vi "A_Read Set Pt Array.vi"(0 "Previous y":dbl, 1 "Period(ms)":dbl, 2 "Result":dbl, 5 "dt":u32, 7 "y array":dbl[](array[numeric]), 12 "arraysize":dbl, 13 "Integral in":dbl) -> (4 "Set Pt Out":dbl, 6 "Integral out":dbl)   [LabVIEW 2011]
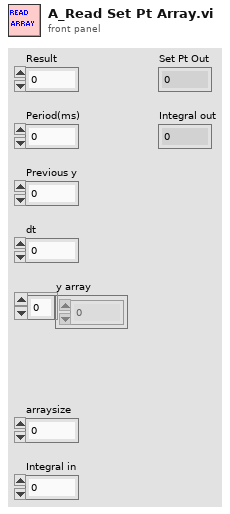
[diagram p1: front panel]
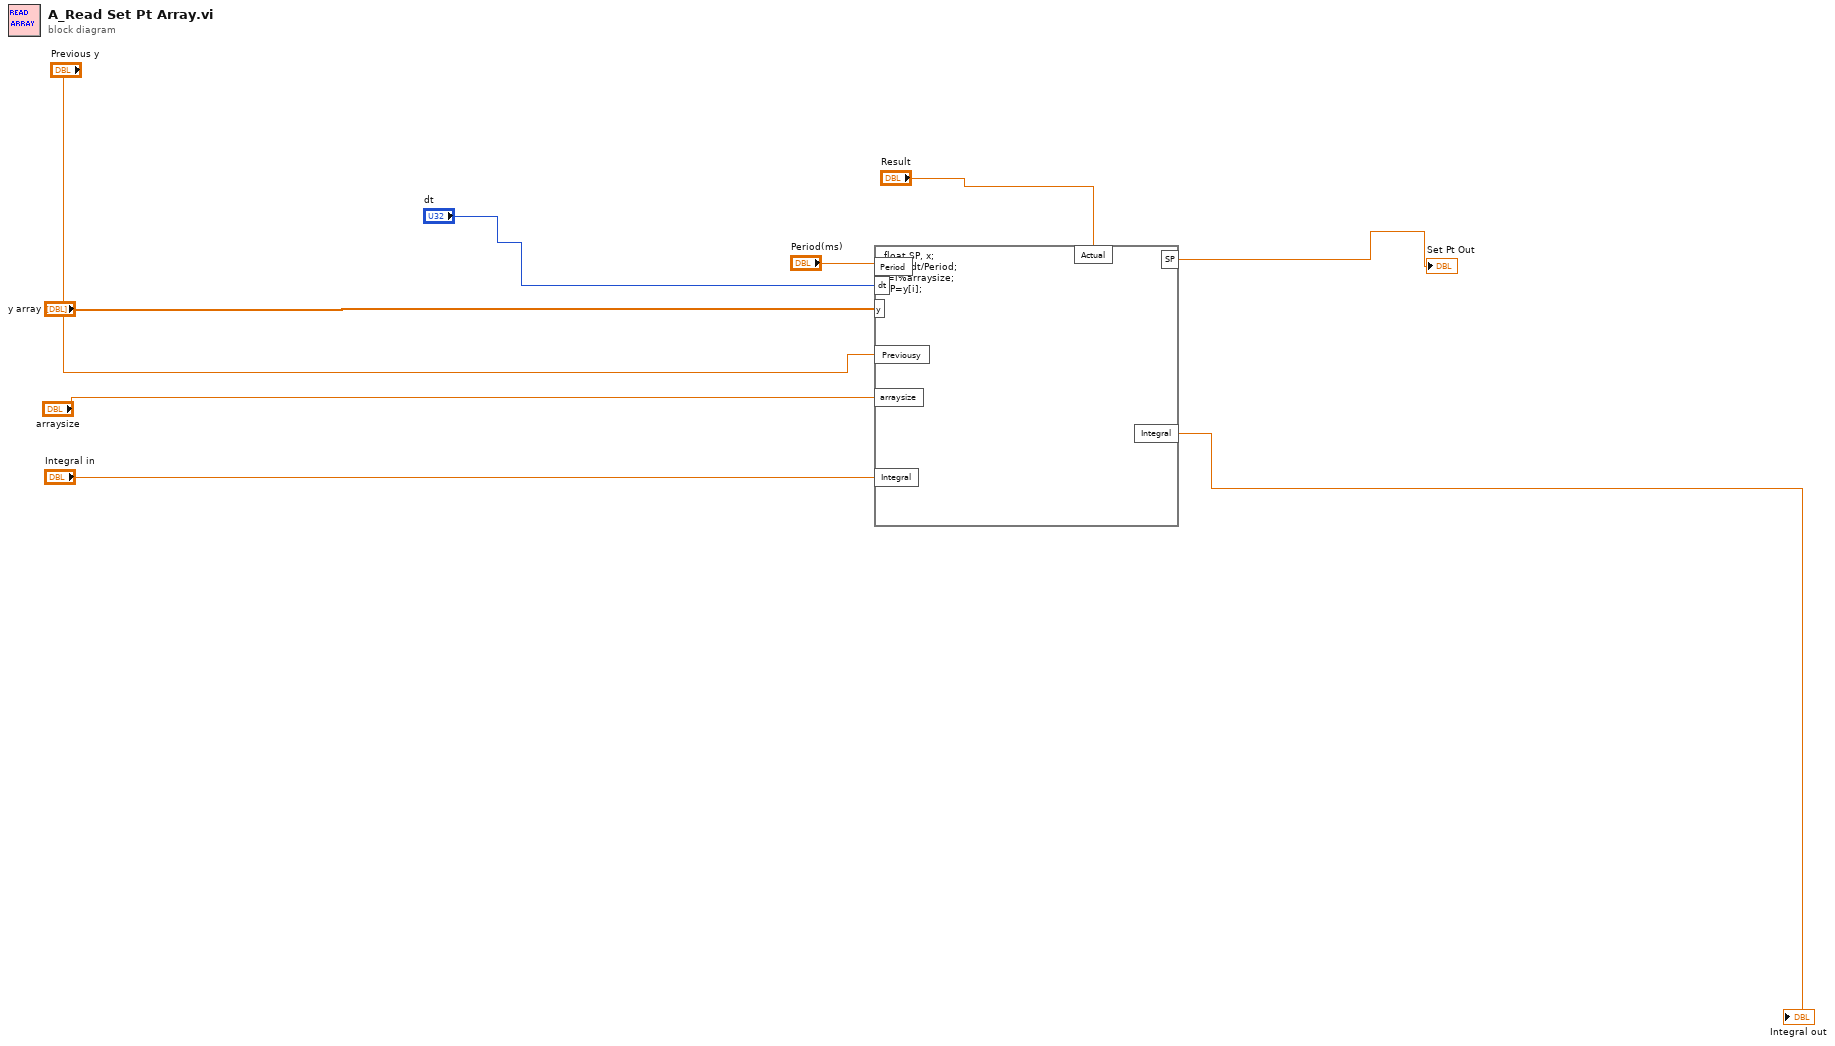
[diagram p0: block diagram]
diagram:
  n1 = formula code="float SP, x;\nint i=dt/Period;\ni=i%arraysize;\nSP=y[i];"("dt"="dt", "Previousy"="Previous y", "y"="y array", "arraysize"="arraysize", "Period"="Period(ms)", "Actual"="Result", "Integral"="Integral in") -> ("SP"=→"Set Pt Out":dbl, "Integral"=→"Integral out":dbl)
